vi "Create Map from Message Indexes to Tx Write Info.vi"(8 "error in":errorcluster, 10 "hardware handles":T1, 11 "1553 channels":T2[](array[typedef])) -> (0 "error out":errorcluster, 3 "map from message indexes to Tx write info":T9)   [LabVIEW 2020, in "Ballard MIL-STD-1553 Engine.lvlib" / "Custom Device.lvlib"]
uses:
  Custom Device.lvlib
  Shared/Map of Message Indexes to Tx Write Info.ctl
  Shared/Tx Write Info.ctl
  Shared/1553 Channel.ctl
  Shared/Terminal Name and Address.ctl
  Shared/Address.ctl
  Shared/Message Definition.ctl
  Shared/Message Type.ctl
  Shared/Terminal Endpoint.ctl
  Shared/Parameter Definition.ctl
  Hardware Handles.ctl
  <instrlib>/BTI1553Lib/BTI1553LV.lvlib
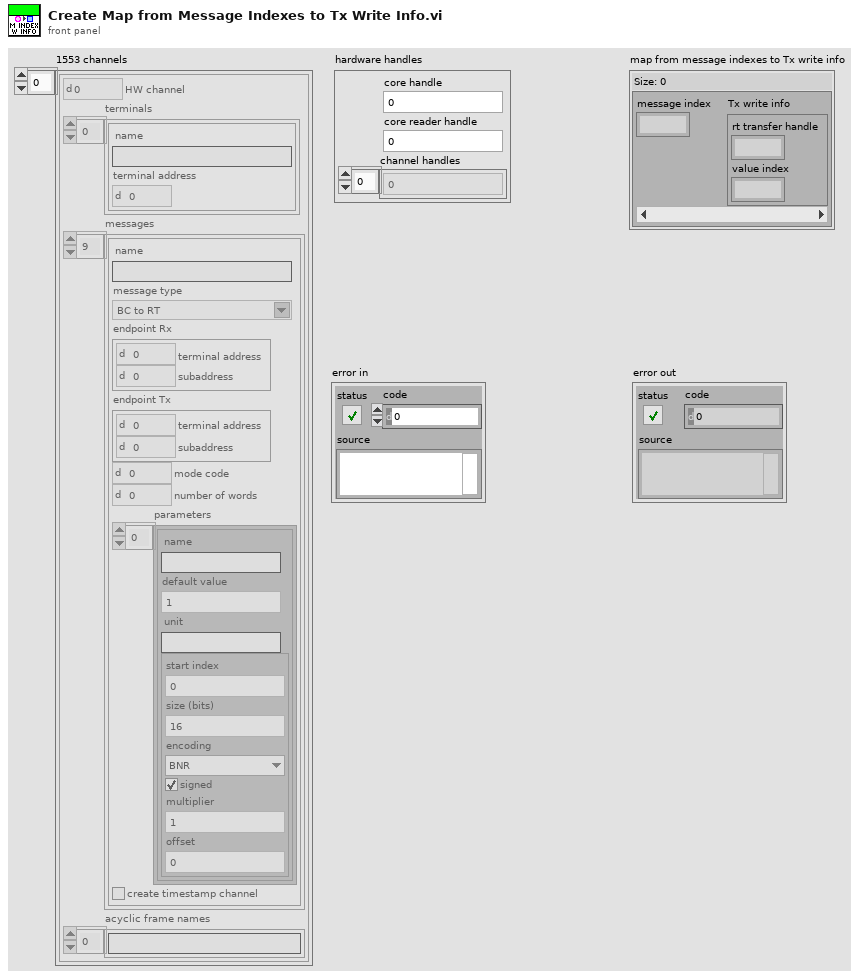
[diagram p1: front panel]
types:
  T1 = typedef "Ballard MIL-STD-1553 Engine.lvlib/Custom Device.lvlib/Hardware Handles.ctl" = cluster{"core handle":u64, "core reader handle":u64, "channel handles":u64[]}
  T2 = typedef "1553 Channel.ctl" = cluster{"HW channel":u16, "terminals":T3[], "messages":T5[], "acyclic frame names":string[]}
  T3 = typedef "Terminal Name and Address.ctl" = cluster{"name":string, "terminal address":T4}
  T4 = typedef "Address.ctl" = u16
  T5 = typedef "Message Definition.ctl" = cluster{"name":string, "message type":T6, "endpoint Rx":T7, "endpoint Tx":T7, "mode code":u16, "number of words":u16, "parameters":cluster{"name":string, "default value":dbl, "unit":string, "parameter definition":T8}[], "create timestamp channel":bool}
  T6 = typedef "Message Type.ctl" = string
  T7 = typedef "Terminal Endpoint.ctl" = cluster{"terminal address":T4, "subaddress":T4}
  T8 = typedef "Parameter Definition.ctl" = cluster{"start index":i32, "size (bits)":i32, "encoding":enum16{"BNR", "BCD", "Discrete"}, "signed":bool, "multiplier":dbl, "offset":dbl}
  T9 = typedef "Map of Message Indexes to Tx Write Info.ctl" = map{i32, T10}
  T10 = typedef "Tx Write Info.ctl" = cluster{"rt transfer handle":u64, "value index":i32}
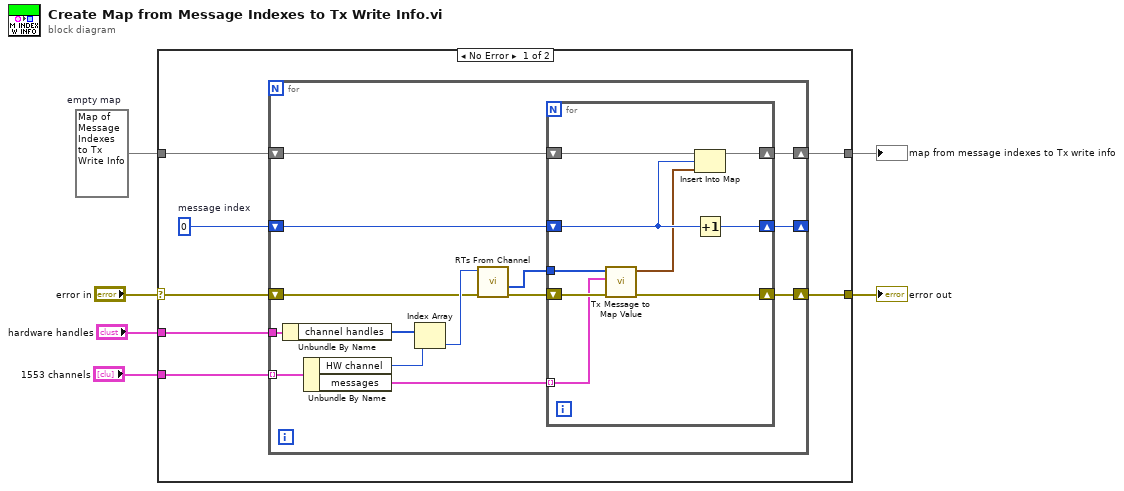
[diagram p0: block diagram]
diagram:
  w4 = T9 {}  # empty map
  n1 = case shown="No Error" "error in" {
    selector: "error in" -> [w8 w37]
    tunnel: "1553 channels" -> [w13 _]
    tunnel: [w12 w38] -> w5
    tunnel: w4 -> [w11 w38]
    tunnel: "hardware handles" -> [w9 _]
    tunnel: [w7 w37] -> w1
    frame No Error {
      w10 = 0  # message index
      n2 = for {
        tunnel: w13 -> [w27] mode=indexing
        shift-right: [w24] -> w12
        shift-left: w11 -> [w26]
        shift-right: [w22] -> _
        shift-left: w10 -> [w23]
        tunnel: w9 -> [w21]
        shift-right: [w14] -> w7
        shift-left: w8 -> [w17]
        n3 = Unbundle By Name(w21) -> ("channel handles"=w20:u64[])
        n4 = Unbundle By Name(w27) -> ("HW channel"=w19:u16, "messages"=w25:T5[])
        n5 = Index Array(array=w20, index=w19) -> (element=w18:u64)
        n6 = call <instrlib>:"RTs From Channel.vi"("error in (no error)"=w17, "channel handle in"=w18) -> ("error out"=w16:errorcluster, "remote terminal handles out"=w15:u64[])  [unwired: 6 in, 2 out]
        n7 = for {
          tunnel: w25 -> [w29] mode=indexing
          shift-right: [w36] -> w24
          shift-left: w26 -> [w35]
          shift-right: [w33] -> w22
          shift-left: w23 -> [w34]
          shift-right: [w31] -> w14
          shift-left: w16 -> [w32]
          tunnel: w15 -> [w30]
          n8 = call "Tx Message to Map Value.vi"("error in"=w32, "message"=w29, "remote terminal handles"=w30) -> ("error out"=w31:errorcluster, "Tx write info"=w28:T10)  [unwired: 7 in]
          n9 = Insert Into Map(map in=w35, key=w34, value=w28) -> (map out=w36:T9)  [unwired: 2 out]
          n10 = Increment(x=w34) -> (x+1=w33:i32)
        }
      }
    }
    frame Error {
    }
  }
  "map from message indexes to Tx write info" <- w5
  "error out" <- w1
